vi "主程序-V1.0.1.vi"() -> (0 "P_ErroInfo_S":string, 1 "P_IsInternal_B":bool, 2 "授权DLL引用输出":refnum<k24>, 3 "Status":T1, 4 "授权通过":bool)   [LabVIEW 2013]
uses:
  AuthorizationToolClassLibrary.dll
panel:
  out "错误输出":errorcluster
  in  "错误输入（无错误）":errorcluster
  out "F_Active_B":bool
  out "F_Simulation_B":bool
  out "F_FloderExsist_B":bool
  # "选择license文件"
  # "F"
  # "T"
  # "F"
  # "F"
  # "T"
  # "T"
  # "默认主板软件版本正确"
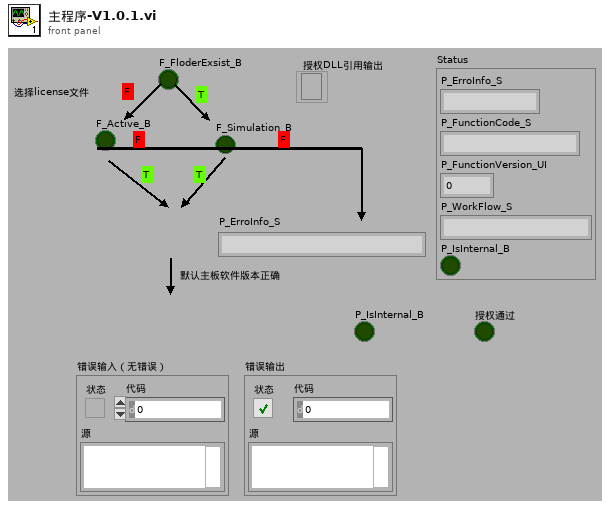
[diagram p1: front panel]
types:
  T1 = cluster{"P_ErroInfo_S":string, "P_FunctionCode_S":string, "P_FunctionVersion_UI":u16, "P_WorkFlow_S":string, "P_IsInternal_B":bool}
  T2 = cluster{"P_ErroInfo_S":string, "P_FunctionCode_S":string, "P_FunctionVersion_UI":u16, "P_FunctionCode_S":string, "P_IsInternal_B":bool}
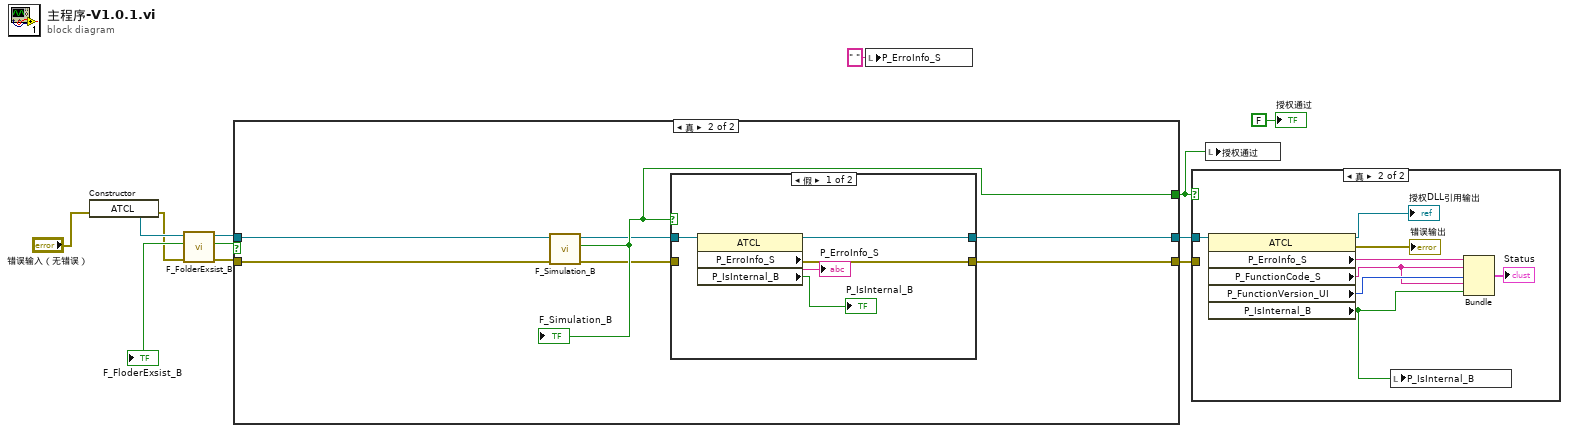
[diagram p0: block diagram]
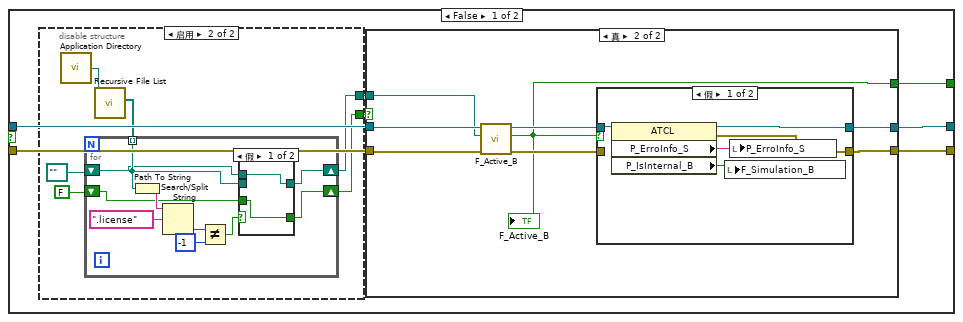
[diagram p3: hidden frame]
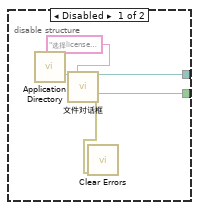
[diagram p4: hidden frame]
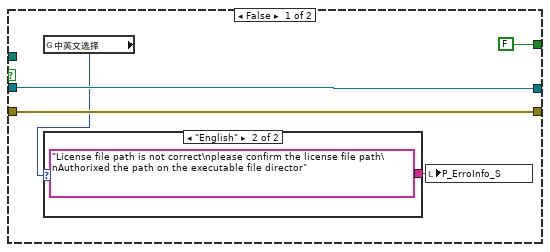
[diagram p6: hidden frame]
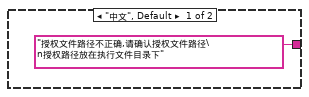
[diagram p7: hidden frame]
diagram:
  n1 = constructor class="ATCL"(error in="错误输入（无错误）") -> (reference out=w5:refnum<k24>, error out=w3:errorcluster)  [unwired: 2 in, 1 out]
  n2 = call "F_FolderExsist_B.vi"("错误输入（无错误）"=w3, "引用"=w5) -> ("错误输出"=w7:errorcluster, "F_FolderExsist_B"=w11:bool, "引用输出"=w8:refnum<k24>)  [unwired: 7 in]
  "F_FloderExsist_B" <- w11
  n3 = case shown="真" w11 {
    tunnel: [w18 w72] -> w1
    tunnel: [w17 w68] -> w9
    tunnel: w8 -> [w16 w71]
    tunnel: w7 -> [w14 w70]
    tunnel: [w15 w67] -> w6
    frame False {
      n4 = disable-structure shown="启用" {
        disable-tunnel: [w21 w24] -> w13
        disable-tunnel: [w20 w26] -> w12
        frame Disabled {
          n5 = call <vilib>:"Application Directory.vi"() -> ("Application Directory"=w23:path)
          n6 = call "文件对话框"("start path"=w23, "prompt"="选择license文件") -> ("selected path"=w20:path, "cancelled"=w21:bool, "error out"=w19:errorcluster)  [unwired: 10 in, 1 out]
          n7 = call <vilib>:"Clear Errors.vi"("error in (no error)"=w19) -> ()  [unwired: 6 in, 1 out]
        }
        frame Enabled {
          n8 = call <vilib>:"Application Directory.vi"() -> ("Application Directory"=w29:path)
          n9 = call <vilib>:"Recursive File List.vi"("Folder Path"=w29) -> ("All Files in Dir"=w28:path[])  [unwired: 6 in, 4 out]
          n10 = for {
            tunnel: w28 -> [w34] mode=indexing
            shift-right: [w33] -> w26
            shift-left: path "" -> [w32]
            shift-right: [w31] -> w24
            shift-left: FALSE -> [w30]
            n11 = Path To String(path=w34) -> (string=w39:string)
            n12 = Search/Split String(string=w39, search string/char (-)=".license" ("搜索字符串/字符(-)")) -> (offset of match=w37:i32)  [unwired: 1 in, 2 out]
            n13 = Not Equal?(x=w37, y=-1) -> (x != y?=w35:bool)
            n14 = case shown="假" w35 {
              selector: w35 -> [_ w42]
              tunnel: w34 -> [_ w43]
              tunnel: [w41 w43] -> w33
              tunnel: w32 -> [w41 _]
              tunnel: [w40 w42] -> w31
              tunnel: w30 -> [w40 _]
              frame False {
              }
              frame True {
              }
            }
          }
        }
      }
      n15 = case shown="真" w13 {
        tunnel: [FALSE w51] -> w18
        tunnel: [w47 w58] -> w17
        tunnel: w16 -> [w48 w56]
        tunnel: [w48 w57] -> w15
        tunnel: w14 -> [w47 w55]
        tunnel: w12 -> [_ w54]
        frame False {
          n16 = global read "中英文全局.vi" "中英文选择"() -> (w44:enum32{"中文", "English"})
          n17 = case shown="\"English\"" w44 {
            tunnel: ["授权文件路径不正确,请确认授权文件路径\n授权路径放在执行文件目录下" ("P_ErroInfo_S") "License file path is not correct\nplease confirm the license file path\nAuthorixed the path on the executable file director" ("P_ErroInfo_S")] -> w45
            frame "中文", Default {
            }
            frame "English" {
            }
          }
          n18 = local write "P_ErroInfo_S"(w45) -> ()
        }
        frame True {
          n19 = call "F_Active_B.vi"("错误输入（无错误）"=w55, "*.license文件路径"=w54, "引用"=w56) -> ("错误输出"=w52:errorcluster, "F_Active_B"=w51:bool, "引用输出"=w53:refnum<k24>)  [unwired: 6 in]
          "F_Active_B" <- w51
          n20 = case shown="假" w51 {
            tunnel: w52 -> [_ w64]
            tunnel: w53 -> [w59 w65]
            tunnel: [w63 w65] -> w57
            tunnel: [w60 w64] -> w58
            frame False {
              n21 = property class="ATCL"(reference=w59) -> (reference out=w63:refnum<k24>, error out=w60:errorcluster, "P_ErroInfo_S"=w62:string, "P_IsInternal_B"=w61:bool)  [unwired: 1 in]
              n22 = local write "F_Simulation_B"(w61) -> ()
              n23 = local write "P_ErroInfo_S"(w62) -> ()
            }
            frame True {
            }
          }
        }
      }
    }
    frame True {
      n24 = call "F_Simulation_B.vi"("错误输入（无错误）"=w70, "引用"=w71) -> ("错误输出"=w69:errorcluster, "F_Simulation_B"=w72:bool, "引用输出"=w66:refnum<k24>)  [unwired: 7 in]
      "F_Simulation_B" <- w72
      n25 = case shown="假" w72 {
        tunnel: w69 -> [_ w79]
        tunnel: [w76 w79] -> w68
        tunnel: [w75 w78] -> w67
        tunnel: w66 -> [w77 w78]
        frame False {
          n26 = property class="ATCL"(reference=w77) -> (reference out=w75:refnum<k24>, error out=w76:errorcluster, "P_ErroInfo_S"=→"P_ErroInfo_S":string, "P_IsInternal_B"=→"P_IsInternal_B":bool)  [unwired: 1 in]
        }
        frame True {
        }
      }
    }
  }
  n27 = local write "P_ErroInfo_S"(" " ("P_ErroInfo_S")) -> ()
  n28 = case shown="真" w1 {
    tunnel: w9 -> [_ _]
    tunnel: w6 -> [_ w86]
    frame False {
    }
    frame True {
      n29 = property class="ATCL"(reference=w86) -> (reference out=→"授权DLL引用输出":refnum<k24>, error out=→"错误输出":errorcluster, "P_ErroInfo_S"=w83:string, "P_FunctionCode_S"=w81:string, "P_FunctionVersion_UI"=w82:u16, "P_IsInternal_B"=w80:bool)  [unwired: 1 in]
      n30 = local write "P_IsInternal_B"(w80) -> ()
      n31 = Bundle("P_ErroInfo_S"=w83, "P_FunctionCode_S"=w81, "P_FunctionVersion_UI"=w82, "P_FunctionCode_S"=w81, "P_IsInternal_B"=w80) -> (→"Status":T2)  [unwired: 1 out]
    }
  }
  n32 = local write "授权通过"(w1) -> ()
  "授权通过" <- FALSE ("授权通过")
